vi "Write Period (ms).vi"(8 "error in (no error)":errorcluster, 10 "Period (ms)":dbl, 11 "Periodic DAQ in":refnum<class "Periodic DAQ.lvclass">=refnum) -> (0 "error out":errorcluster, 3 "Periodic DAQ out":refnum<class "Periodic DAQ.lvclass">)   [LabVIEW 2014, in "Periodic DAQ.lvclass"]
uses:
  Periodic DAQ.lvclass
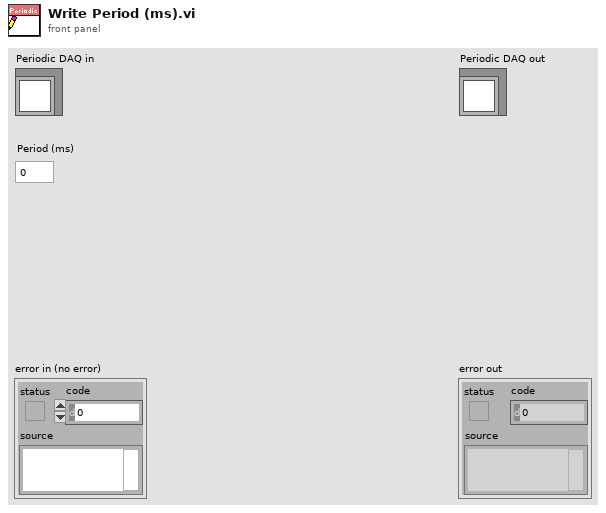
[diagram p1: front panel]
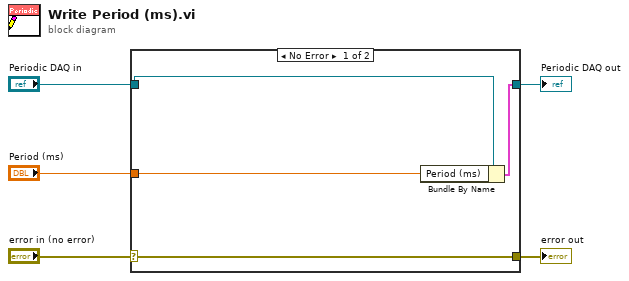
[diagram p0: block diagram]
diagram:
  n1 = case shown="No Error" "error in (no error)" {
    selector: "error in (no error)" -> [w9 w10]
    tunnel: [w9 w10] -> w4
    tunnel: [w7 w11] -> w2
    tunnel: "Periodic DAQ in" -> [w8 w11]
    tunnel: "Period (ms)" -> [w6 _]
    frame No Error {
      n2 = Bundle By Name(cluster=w8, "Period (ms)"=w6) -> (w7:cluster{})
    }
    frame Error {
    }
  }
  "error out" <- w4
  "Periodic DAQ out" <- w2
